vi "OC200_Test.vi"() -> ()   [LabVIEW 2019]
panel:
  out "pressure":dbl
  in  "device_addr":u8=22
  out "response":string
  in  "port":u16=4196
  in  "ip_addr":string="192.168.24.133"
  out "time":timestamp format="%<%Y-%m-%d %H:%M:%S>T"
  out "status":bool
  in  "wait (ms)":u32=1000
  in  "stop":bool
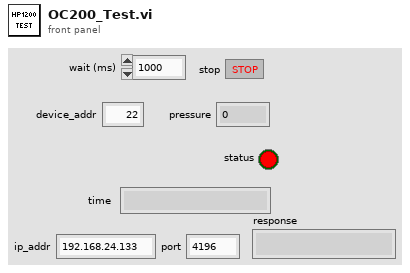
[diagram p1: front panel]
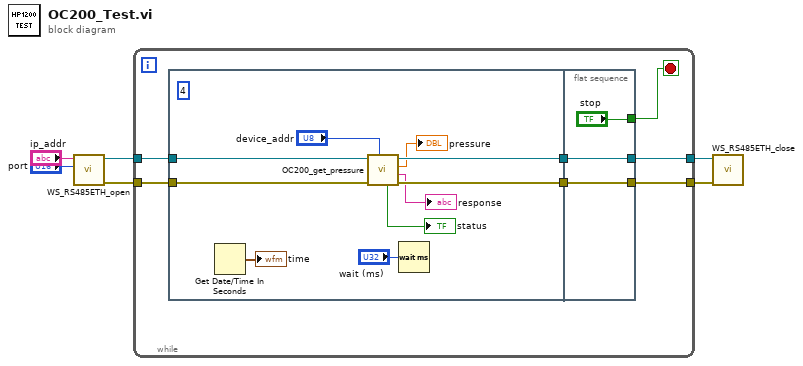
[diagram p0: block diagram]
diagram:
  n1 = call "WS_RS485ETH_open.vi"("port"="port", "ip_addr"="ip_addr") -> ("error out"=w4:errorcluster, "conn_id"=w6:refnum<k5>)  [unwired: 7 in, 1 out]
  n2 = while {
    tunnel: w6 -> [w12]
    tunnel: [w10] -> w5
    tunnel: w4 -> [w9]
    tunnel: [w7] -> w3
    stop <- w13 stop-if-true
    n3 = flat-sequence {
      tunnel: w12 -> [w23]
      tunnel: [w22] -> w11
      tunnel: w9 -> [w21]
      tunnel: [w20] -> w8
      tunnel: ["stop"] -> w13
      tunnel: w11 -> [w25]
      tunnel: [w25] -> w10
      tunnel: w8 -> [w24]
      tunnel: [w24] -> w7
      frame #0 {
        (unwired) 4
        n4 = Get Date/Time In Seconds() -> (seconds since 1Jan1904=→"time":timestamp)
        n5 = call "OC200_get_pressure.vi"("device_addr"="device_addr", "error in"=w21, "conn_id_in"=w23) -> ("error out"=w20:errorcluster, "response"=→"response":string, "pressure"=→"pressure":dbl, "conn_id_out"=w22:refnum<k5>, "status"=→"status":bool)  [unwired: 4 in]
        n6 = Wait (ms)(milliseconds to wait="wait (ms)") -> ()  [unwired: 1 out]
      }
      frame #1 {
      }
    }
  }
  n7 = call "WS_RS485ETH_close.vi"("error in"=w3, "conn_id"=w5) -> ()  [unwired: 8 in, 2 out]
